vi "ssh2_echo.vi"() -> ()   [LabVIEW 2017]
doc: "Illustrates how to echo data from an SSH server using the 'cat' utility."
uses:
  libssh2/libssh2_session_handshake_tcp.vi
  libssh2/Wait Socket (TCP).vi
  libssh2/libssh2_init_default.vi
  libssh2/libssh2_session_init_ex.vi
  <vilib>/Utility/tcp.llb/TCP Get Raw Net Object.vi
  libssh2/libssh2_session_handshake_socket.vi
  libssh2/libssh2_userauth_password_ex.vi
  libssh2/libssh2_channel_open_ex.vi
  libssh2/libssh2_channel_process_startup.vi
  libssh2/Wait Socket (Socket).vi
  libssh2/libssh2_channel_write_ex.vi
  libssh2/libssh2_channel_read_ex.vi
  libssh2/libssh2.lvlib
panel:
  out "Numeric":i32
  out "read buffer size":i32
  out "read buffer":string
  in  "password":string
  in  "username":string
  in  "hostname":string="localhost"
  out "error out":errorcluster
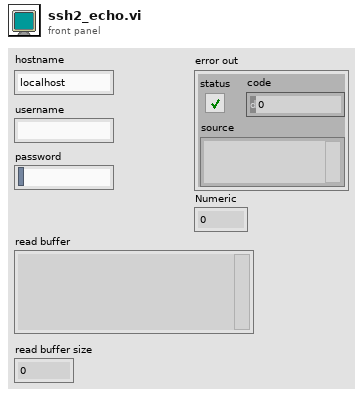
[diagram p1: front panel]
types:
  T1 = typedef "libssh2.lvlib/Session Refnum.ctl" = refnum<k1>
  T2 = typedef "libssh2.lvlib/Channel Refnum.ctl" = refnum<k1>
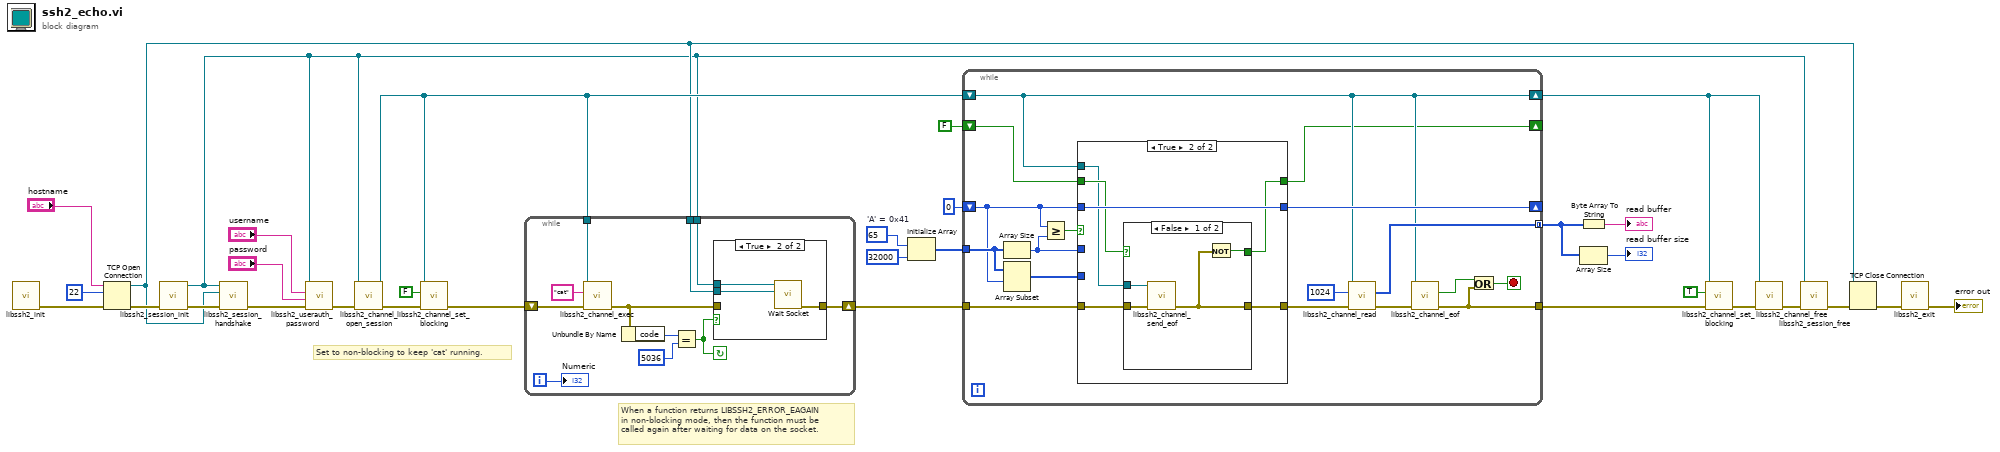
[diagram p0: block diagram]
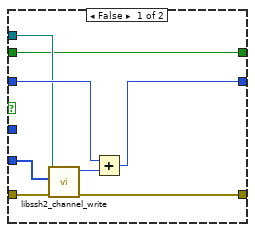
[diagram p3: hidden frame]
diagram:
  w13 = u8 65  # 'A' = 0x41
  # "When a function returns LIBSSH2_ERROR_EAGAIN\nin non-blocking mode, then the function must be\ncalled again after waiting for data on the socket."
  # "Set to non-blocking to keep 'cat' running."
  n1 = call-poly "libssh2_init.vi"() -> ("error out"=w32:errorcluster)  [unwired: 11 in]
  n2 = TCP Open Connection(address="hostname", remote port or service name=u16 22, error in (no error)=w32) -> (connection ID=w2:refnum<k5>, error out=w6:errorcluster)  [unwired: 2 in]
  n3 = call "libssh2_session_init.vi"("error in (no error)"=w6) -> ("error out"=w27:errorcluster, "session"=w1:T1)  [unwired: 9 in]
  n4 = call-poly "libssh2_session_handshake.vi"("error in (no error)"=w27, "tcp connection"=w2, "session"=w1) -> ("error out"=w26:errorcluster)  [unwired: 8 in]
  n5 = call "libssh2_userauth_password.vi"("error in (no error)"=w26, "password"="password", "username"="username", "session"=w1) -> ("error out"=w25:errorcluster)  [unwired: 7 in]
  n6 = call "libssh2_channel_open_session.vi"("error in (no error)"=w25, "session"=w1) -> ("error out"=w22:errorcluster, "channel"=w5:T2)  [unwired: 8 in]
  n7 = call "libssh2_channel_set_blocking.vi"("error in (no error)"=w22, "blocking"=FALSE, "channel"=w5) -> ("error out"=w19:errorcluster)  [unwired: 8 in]
  n8 = while {
    tunnel: w5 -> [w41]
    shift-right: [w37] -> w3
    shift-left: w19 -> [w43]
    tunnel: w2 -> [w35]
    tunnel: w1 -> [w34]
    i -> [w33]
    stop <- w38 continue-if-true
    n9 = call "libssh2_channel_exec.vi"("error in (no error)"=w43, "command"="cat", "channel"=w41) -> ("error out"=w36:errorcluster)  [unwired: 8 in]
    n10 = Unbundle By Name(w36) -> ("code"=w40:i32)
    n11 = Equal?(x=w40, y=5036) -> (x = y?=w38:bool)
    n12 = case shown="True" w38 {
      tunnel: [w44 w47] -> w37
      tunnel: w36 -> [w44 _]
      tunnel: w35 -> [_ w45]
      tunnel: w34 -> [_ w46]
      frame False {
      }
      frame True {
        n13 = call-poly "Wait Socket.vi"("tcp connection"=w45, "session"=w46) -> ("error out"=w47:errorcluster)  [unwired: 9 in]
      }
    }
    "Numeric" <- w33
  }
  n14 = Initialize Array(w13, 32000 ("dimension size")) -> (w14:u8[])
  n15 = while {
    tunnel: [w55] -> w9
    tunnel: w3 -> [w64]
    tunnel: w14 -> [w62]
    shift-right: [w61] -> _
    shift-left: 0 -> [w59]
    tunnel: [w56] -> w8 mode=concatenating
    shift-right: [w53] -> w4
    shift-left: w5 -> [w53]
    shift-right: [w49] -> _
    shift-left: FALSE -> [w50]
    stop <- w60 stop-if-true
    n16 = Array Size(array=w62) -> (size(s)=w52:i32)
    n17 = Array Subset(array=w62, index=w59) -> (w63:u8[])  [unwired: 1 in]
    n18 = Greater Or Equal?(x=w59, y=w52) -> (x >= y?=w58:bool)
    n19 = case shown="True" w58 {
      tunnel: w64 -> [w72 w77]
      tunnel: [w65 w76] -> w51
      tunnel: w53 -> [w69 w74]
      tunnel: w63 -> [w67 _]
      tunnel: [w68 w78] -> w61
      tunnel: w59 -> [w70 w78]
      tunnel: w52 -> [_ _]
      tunnel: w50 -> [w66 w75]
      tunnel: [w66 w73] -> w49
      frame False {
        n20 = call "libssh2_channel_write.vi"("error in (no error)"=w72, "buffer"=w67, "channel"=w69) -> ("error out"=w65:errorcluster, "bytes written"=w71:i32)  [unwired: 7 in]
        n21 = Add(x=w70, y=w71) -> (x+y=w68:i32)
      }
      frame True {
        n22 = case shown="False" w75 {
          selector: w75 -> [_ w83]
          tunnel: w77 -> [w82 w84]
          tunnel: [w79 w84] -> w76
          tunnel: w74 -> [w81 _]
          tunnel: [w80 w83] -> w73
          frame False {
            n23 = call "libssh2_channel_send_eof.vi"("error in (no error)"=w82, "channel"=w81) -> ("error out"=w79:errorcluster)  [unwired: 9 in]
            n24 = Not(x=w79) -> (.not. x?=w80:bool)
          }
          frame True {
          }
        }
      }
    }
    n25 = call "libssh2_channel_read.vi"("error in (no error)"=w51, "buffer length"=1024, "channel"=w53) -> ("error out"=w48:errorcluster, "buffer"=w56:u8[])  [unwired: 7 in]
    n26 = call "libssh2_channel_eof.vi"("error in (no error)"=w48, "channel"=w53) -> ("error out"=w55:errorcluster, "eof"=w54:bool)  [unwired: 8 in]
    n27 = Or(x=w54, y=w55) -> (x .or. y?=w60:bool)
  }
  n28 = Byte Array To String(unsigned byte array=w8) -> (string=→"read buffer":string)
  n29 = Array Size(array=w8) -> (size(s)=→"read buffer size":i32)
  n30 = call "libssh2_channel_set_blocking.vi"("error in (no error)"=w9, "blocking"=TRUE, "channel"=w4) -> ("error out"=w16:errorcluster)  [unwired: 8 in]
  n31 = call "libssh2_channel_free.vi"("error in (no error)"=w16, "channel"=w4) -> ("error out"=w20:errorcluster)  [unwired: 9 in]
  n32 = call "libssh2_session_free.vi"("error in (no error)"=w20, "session"=w1) -> ("error out"=w21:errorcluster)  [unwired: 9 in]
  n33 = TCP Close Connection(connection ID=w2, error in (no error)=w21) -> (error out=w29:errorcluster)  [unwired: 1 in, 1 out]
  n34 = call "libssh2_exit.vi"("error in (no error)"=w29) -> ("error out"=→"error out":errorcluster)  [unwired: 10 in]
